vi "Database Alter Table Set Field Constraint Unique.vi"(8 "error in (no error)":errorcluster, 9 "Field (\"\")":string, 10 "Table (\"\")":string, 11 "Connection Refnum":T1) -> (0 "error out":errorcluster, 3 "Connection Refnum":T1)   [LabVIEW 2011]
uses:
  SI.LIB/ODBC/SQL Controls/Connection Refnum.ctl
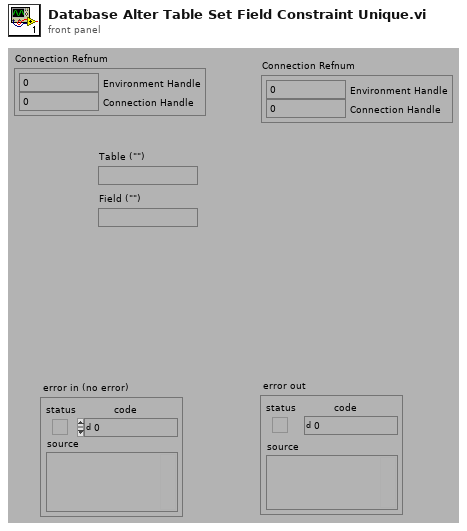
[diagram p1: front panel]
types:
  T1 = typedef "Connection Refnum.ctl" = cluster{"Environment Handle":i32, "Connection Handle":i32}
  T2 = typedef "Statement Refnum.ctl" = cluster{"Statement Handle":i32, "Parameter Number":u16}
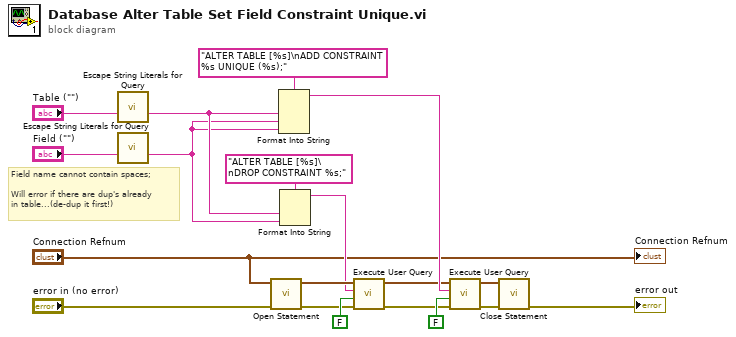
[diagram p0: block diagram]
diagram:
  # "Field name cannot contain spaces;\n\nWill error if there are dup's already\nin table...(de-dup it first!)"
  n1 = call "Escape String Literals for Query.vi"("String"="Table (\"\")") -> ("escaped String"=w6:string)  [unwired: 1 in, 13 out]
  n2 = call "Escape String Literals for Query.vi"("String"="Field (\"\")") -> ("escaped String"=w5:string)  [unwired: 1 in, 13 out]
  n3 = call "Open Statement.vi"("error in (no error)"="error in (no error)", "Connection Refnum"="Connection Refnum") -> ("error out"=w11:errorcluster, "Statement Refnum"=w10:T2)  [unwired: 4 out]
  n4 = Format Into String(format string="ALTER TABLE [%s]\nADD CONSTRAINT %s UNIQUE (%s);" ("User Query"), w6, w5, w5) -> (resulting string=w15:string)  [unwired: 2 in, 1 out]
  n5 = Format Into String(format string="ALTER TABLE [%s]\nDROP CONSTRAINT %s;" ("User Query"), w6, w5) -> (resulting string=w4:string)  [unwired: 2 in, 1 out]
  n6 = call "Execute User Query.vi"("error in (no error)"=w11, "Return Data? (f)"=FALSE, "User Query"=w4, "Statement Refnum"=w10) -> ("error out"=w8:errorcluster, "Statement Refnum"=w9:T2)  [unwired: 2 out]
  n7 = call "Execute User Query.vi"("error in (no error)"=w8, "Return Data? (f)"=FALSE, "User Query"=w15, "Statement Refnum"=w9) -> ("error out"=w18:errorcluster, "Statement Refnum"=w17:T2)  [unwired: 2 out]
  n8 = call "Close Statement.vi"("error in (no error)"=w18, "Statement Refnum"=w17) -> ("error out"=→"error out":errorcluster)  [unwired: 5 out]
  "Connection Refnum" <- "Connection Refnum"
